vi "KISSIA_TO ARRAY_SET_4VIAS.vi"(10 "String":string="SET Valvula 4VIAS: 1 y pausa 0.1s") -> (1 "Array":string[](array[string]))   [LabVIEW 2017]
panel:
  # "SET Valvula 4VIAS: 1 y pausa 0.1s"
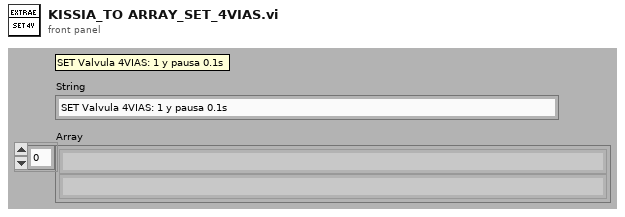
[diagram p1: front panel]
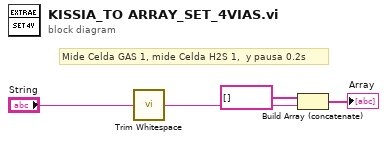
[diagram p0: block diagram]
diagram:
  # "Mide Celda GAS 1, mide Celda H2S 1,  y pausa 0.2s"
  n1 = call <vilib>:"Trim Whitespace.vi"("string"="String") -> ("trimmed string"=w1:string)  [unwired: 1 in]
  n2 = Build Array (concatenate)(string[] [] ("Array I"), w1) -> (→"Array":string[])
